vi "Initiate Stream.vi"(0 "niUsrpRio Session":T1={"FPGA Interface"=refnum, "RIO Interface Number"=0, "Data Clock Rate"=0, "FPGA Data Clock Rate"=0, "Global Settings Register Bus"=refnum, "Radio 0 Settings Register Bus"=refnum, "Radio 1 Settings Register Bus"=refnum, "Radio Settings Bus Semaphore"=refnum, "DB Queues"=[], "Characterization Data Valid?"=FALSE, "EEPROM Header"={"Checksum"=0, "Product Code"=0, "Hardware Current Version"=0, "Hardware Oldest Compatible Version"=0, "EEPROM Map Current Version"=0, "EEPROM Map Oldest Compatible Version"=0, "User Password"="", "Pointer to Factory Header"=0, "Pointer to User Header"=0, "Recommended Interval"=0, "Number of Reserved Bytes"=9, "Number of Daughterboards"=0, "Daughterboard IDs"=[], "Daughterboard Serial Numbers"=[]}, "Device Data Header"={"Checksum"=0, "Number of Channels"=0, "Number of Gain Settings"=[], "Pointer to Characterization Data"=[], "Number of Reserved Bytes"=27, "Number of Frequencies"=[]}, "EEPROM Characterization Header"={"Checksum"=0, "Date"=timestamp(0 s since 1904-01-01), "Temperature"=0.0, "Misc. Info"="", "Pointer to Device Data Header"=0, "Number of Reserved Bytes"=28}, "Characterization Data"=[], "FPGA Current Version"=0, "FPGA Oldest Compatible Version"=0, "Fixed Logic Current Version"=0, "Fixed Logic Oldest Compatible Version"=0, "FPGA Radio Settings Bus Current Version"=0, "FPGA Radio Settings Bus Oldest Compatible Version"=0, "FPGA Board Config Current Version"=0, "FPGA Board Config Oldest Compatible Version"=0, "Daughterboard Clock Rate"=0, "daughterboard configuration session handles"=[]} {"Daughterboard Clock Rate" format="%#.3pHz"; "FPGA Data Clock Rate" format="%#.3pHz"; "Data Clock Rate" format="%#.3pHz"; "Characterization Data"."Frequencies [Hz]" format="%#_6p"; "EEPROM Characterization Header"."Pointer to Device Data Header" format="%x"; "EEPROM Characterization Header"."Checksum" format="%x"; "Device Data Header"."Pointer to Characterization Data" format="%x"; "Device Data Header"."Checksum" format="%x"; "EEPROM Header"."Pointer to User Header" format="%x"; "EEPROM Header"."Pointer to Factory Header" format="%x"; "EEPROM Header"."Product Code" format="%x"; "EEPROM Header"."Checksum" format="%x"}, 1 "scope":string(combo)="rx", 11 "error in":errorcluster) -> (4 "niUsrpRio Session (out)":T1={"FPGA Interface"=refnum, "RIO Interface Number"=0, "Data Clock Rate"=0, "FPGA Data Clock Rate"=0, "Global Settings Register Bus"=refnum, "Radio 0 Settings Register Bus"=refnum, "Radio 1 Settings Register Bus"=refnum, "Radio Settings Bus Semaphore"=refnum, "DB Queues"=[], "Characterization Data Valid?"=FALSE, "EEPROM Header"={"Checksum"=0, "Product Code"=0, "Hardware Current Version"=0, "Hardware Oldest Compatible Version"=0, "EEPROM Map Current Version"=0, "EEPROM Map Oldest Compatible Version"=0, "User Password"="", "Pointer to Factory Header"=0, "Pointer to User Header"=0, "Recommended Interval"=0, "Number of Reserved Bytes"=9, "Number of Daughterboards"=0, "Daughterboard IDs"=[], "Daughterboard Serial Numbers"=[]}, "Device Data Header"={"Checksum"=0, "Number of Channels"=0, "Number of Gain Settings"=[], "Pointer to Characterization Data"=[], "Number of Reserved Bytes"=27, "Number of Frequencies"=[]}, "EEPROM Characterization Header"={"Checksum"=0, "Date"=timestamp(0 s since 1904-01-01), "Temperature"=0.0, "Misc. Info"="", "Pointer to Device Data Header"=0, "Number of Reserved Bytes"=28}, "Characterization Data"=[], "FPGA Current Version"=0, "FPGA Oldest Compatible Version"=0, "Fixed Logic Current Version"=0, "Fixed Logic Oldest Compatible Version"=0, "FPGA Radio Settings Bus Current Version"=0, "FPGA Radio Settings Bus Oldest Compatible Version"=0, "FPGA Board Config Current Version"=0, "FPGA Board Config Oldest Compatible Version"=0, "Daughterboard Clock Rate"=0, "daughterboard configuration session handles"=[]} {"Daughterboard Clock Rate" format="%#.3pHz"; "FPGA Data Clock Rate" format="%#.3pHz"; "Data Clock Rate" format="%#.3pHz"; "Characterization Data"."Frequencies [Hz]" format="%#_6p"; "EEPROM Characterization Header"."Pointer to Device Data Header" format="%x"; "EEPROM Characterization Header"."Checksum" format="%x"; "Device Data Header"."Pointer to Characterization Data" format="%x"; "Device Data Header"."Checksum" format="%x"; "EEPROM Header"."Pointer to User Header" format="%x"; "EEPROM Header"."Pointer to Factory Header" format="%x"; "EEPROM Header"."Product Code" format="%x"; "EEPROM Header"."Checksum" format="%x"}, 15 "error out":errorcluster)   [LabVIEW 2020]
doc: "Initiates the stream. This is required before you acquire/generate data with the Fetch Rx Data or Write Tx Data VIs. Initiation includes resetting the Rx/Tx streams and the DSP.\n\n<b>Multi-device usage:</b>\nInitiate the master device last, after initiating all the slave devices.\n\n<B>Input Parameters</B>\n\n<B>niUsrpRio Session</B> is the object created by the Open VI and used as the session handle for the USRP RIO design library.\n\n<B>scope</B> is the channel on which stream is to be initiated. The options are \"rx/RF 0\", \"rx/RF 1\", \"tx/RF 0\", and \"tx/RF 1\".\n\n<B>error in</B> describes error conditions that occur before this node runs. This input provides standard 'error in' functionality.\n\n<B>Output Parameters</B>\n\n<B>niUsrpRio Session (out)</B> is the niUsrpRio session used in all subsequent USRP RIO design library host VIs.\n\n<B>error out</B> contains error information. This output provides standard 'error out' functionality."
uses:
  <instrlib>/niUsrpRio/Config/v1/Host/Public/niUsrpRio Session.ctl
  <instrlib>/_niInstr/Register Bus/v0/Host/Public/Register Bus Session.ctl
  <instrlib>/_niInstr/Register Bus/v0/Host/Private/Session Data.ctl
  <instrlib>/niUsrpRio/Config/v1/Host/Private/DB Queue Reference.ctl
  <instrlib>/niUsrpRio/Config/v1/Host/Private/Daughterboard Data.ctl
  <instrlib>/niUsrpRio/Config/v1/Host/Private/ATR state data.ctl
  <instrlib>/niUsrpRio/Config/v1/Host/Private/Antenna Configuration.ctl
  <instrlib>/niUsrpRio/Config/v1/Host/Private/CPLD Power Mode.ctl
  <instrlib>/niUsrpRio/Config/v1/Host/Public/EEPROM Header.ctl
  <instrlib>/niUsrpRio/Config/v1/Host/Public/EEPROM Device Data Header.ctl
  <instrlib>/niUsrpRio/Config/v1/Host/Public/EEPROM Characterization Header.ctl
  <instrlib>/niUsrpRio/Config/v1/Host/Public/Characterization Data.ctl
  <instrlib>/niUsrpRio/Config/v1/Host/Public/IQ Imbalance.ctl
  Streaming Xvcr FPGA Ref.ctl
  <vilib>/Utility/error.llb/Error Cluster From Error Code.vi
  <vilib>/rvi/errors/niLvFpgaAdjustHostInterfaceError.vi
  <vilib>/ErrorRing/Error Ring.xnode
  <vilib>/rvi/interface/nirviReadWriteControl/nirviReadWriteControl.xnode
  <vilib>/rvi/interface/Simulation/niFpgaSimulationCallBeginRW.vi
  NiFpgaLv.dll
  <instrlib>/niUsrpRio/Config/v1/Host/niUsrpRio Config v1 Host.lvlib
  <instrlib>/_niInstr/Register Bus/v0/Host/niInstr Register Bus v0 Host.lvlib
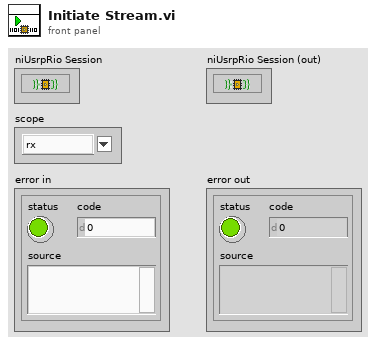
[diagram p1: front panel]
types:
  T1 = typedef "niUsrpRio Config v1 Host.lvlib/niUsrpRio Session.ctl" = cluster{"FPGA Interface":refnum<k20>, "RIO Interface Number":u32, "Data Clock Rate":u32, "FPGA Data Clock Rate":u32, "Global Settings Register Bus":T2, "Radio 0 Settings Register Bus":T2, "Radio 1 Settings Register Bus":T2, "Radio Settings Bus Semaphore":T3, "DB Queues":T4[], "Characterization Data Valid?":bool, "EEPROM Header":T5, "Device Data Header":T6, "EEPROM Characterization Header":T7, "Characterization Data":T8[], "FPGA Current Version":u32, "FPGA Oldest Compatible Version":u32, "Fixed Logic Current Version":u32, "Fixed Logic Oldest Compatible Version":u32, "FPGA Radio Settings Bus Current Version":u32, "FPGA Radio Settings Bus Oldest Compatible Version":u32, "FPGA Board Config Current Version":u32, "FPGA Board Config Oldest Compatible Version":u32, "Daughterboard Clock Rate":u32, "daughterboard configuration session handles":u64[]}
  T2 = typedef "niInstr Register Bus v0 Host.lvlib/Register Bus Session.ctl" = refnum<queue>
  T3 = typedef "Semaphore RefNum" = refnum<k1>
  T4 = typedef "niUsrpRio Config v1 Host.lvlib/DB Queue Reference.ctl" = refnum<queue>
  T5 = typedef "niUsrpRio Config v1 Host.lvlib/EEPROM Header.ctl" = cluster{"Checksum":u32, "Product Code":u16, "Hardware Current Version":u16, "Hardware Oldest Compatible Version":u16, "EEPROM Map Current Version":u16, "EEPROM Map Oldest Compatible Version":u16, "User Password":string, "Pointer to Factory Header":u32, "Pointer to User Header":u32, "Recommended Interval":u16, "Number of Reserved Bytes":i32, "Number of Daughterboards":u8, "Daughterboard IDs":u16[], "Daughterboard Serial Numbers":string[]}
  T6 = typedef "niUsrpRio Config v1 Host.lvlib/EEPROM Device Data Header.ctl" = cluster{"Checksum":u32, "Number of Channels":u8, "Number of Gain Settings":u16[], "Pointer to Characterization Data":u32[], "Number of Reserved Bytes":i32, "Number of Frequencies":u16[]}
  T7 = typedef "niUsrpRio Config v1 Host.lvlib/EEPROM Characterization Header.ctl" = cluster{"Checksum":u32, "Date":timestamp, "Temperature":sgl, "Misc. Info":string, "Pointer to Device Data Header":u32, "Number of Reserved Bytes":i32}
  T8 = typedef "niUsrpRio Config v1 Host.lvlib/Characterization Data.ctl" = cluster{"Gains[dB]":dbl[], "Frequencies [Hz]":dbl[], "IQ Imbalance Table":T9[], "Measured Gains[dB]":dbl[][]}
  T9 = typedef "niUsrpRio Config v1 Host.lvlib/IQ Imbalance.ctl" = cluster{"Gain Imbalance [linear]":dbl, "Phase Imbalance [radians]":dbl, "Offset":cdb}
  T10 = typedef "Streaming Xvcr FPGA Ref.ctl" = refnum<k20>
  T11 = typedef "niUsrpRio Config v1 Host.lvlib/Device Subfunction.ctl" = enum16{"rx", "tx", "all"}
  T12 = typedef "niUsrpRio Config v1 Host.lvlib/RF Channel 2.ctl" = enum16{"0", "1", "2", "3", "All"}
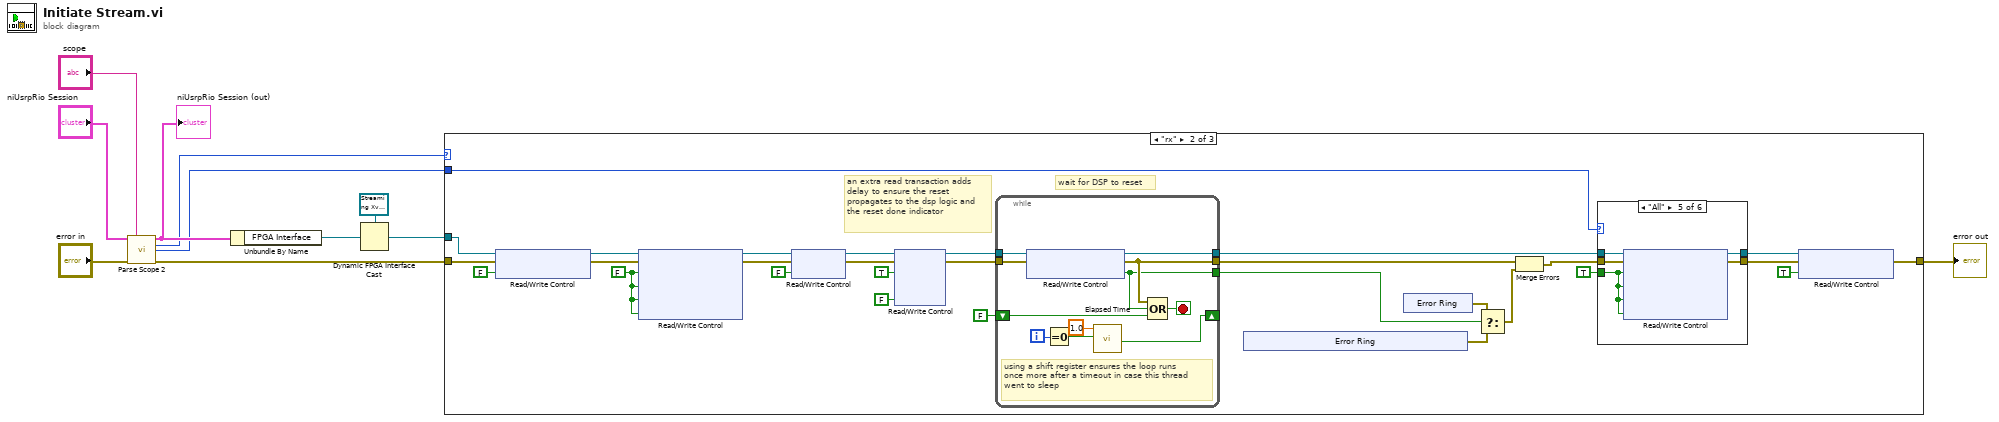
[diagram p0: block diagram]
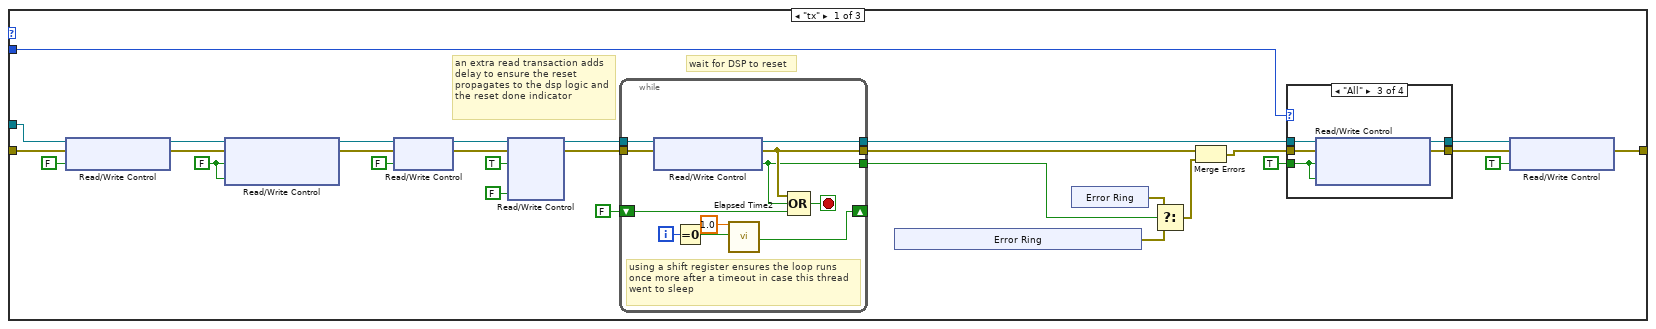
[diagram p2: hidden frame]
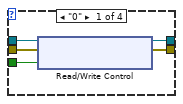
[diagram p3: hidden frame]
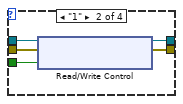
[diagram p4: hidden frame]
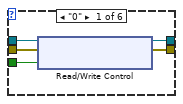
[diagram p6: hidden frame]
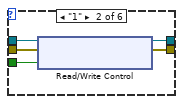
[diagram p7: hidden frame]
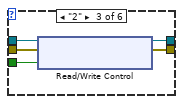
[diagram p8: hidden frame]
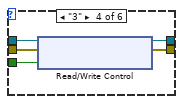
[diagram p9: hidden frame]
diagram:
  n1 = call <instrlib>:"Parse Scope 2.vi"("niUsrpRio Session"="niUsrpRio Session", "scope"="scope", "error in"="error in") -> ("niUsrpRio Session (out)"=w11:T1, "Device Subfunction"=w8:T11, "Device Subfunction Channel"=w7:T12, "error out"=w6:errorcluster)  [unwired: 4 in, 5 out]
  "niUsrpRio Session (out)" <- w11
  n2 = Unbundle By Name(w11) -> ("FPGA Interface"=w4:refnum<k20>)
  n3 = Dynamic FPGA Interface Cast(Session In=T10 refnum ("Type"), Type=w4) -> (Session Out=w3:T10)
  n4 = case shown="\"rx\"" w8 {
    tunnel: w3 -> [w24 w85 _]
    tunnel: [w25 w86 w148] -> w2
    tunnel: w6 -> [w31 w92 w148]
    tunnel: w7 -> [w32 w93 _]
    frame "tx" {
      w12 = FALSE ("tx 0.stream enable")
      # "an extra read transaction adds delay to ensure the reset propagates to the dsp logic and the reset done indicator"
      # "wait for DSP to reset"
      n5 = xnode "Read/Write Control"("FPGA VI Reference In"=w24, "error in"=w31, "tx.trigger enable"=FALSE) -> ("FPGA VI Reference Out"=w29:T10, "error out"=w30:errorcluster)
      n6 = xnode "Read/Write Control"("FPGA VI Reference In"=w29, "error in"=w30, "tx 0.stream enable"=w12, "tx 1.stream enable"=w12) -> ("FPGA VI Reference Out"=w35:T10, "error out"=w36:errorcluster)
      n7 = xnode "Read/Write Control"("FPGA VI Reference In"=w35, "error in"=w36, "tx.abort"=FALSE) -> ("FPGA VI Reference Out"=w18:T10, "error out"=w17:errorcluster)
      n8 = xnode "Read/Write Control"("FPGA VI Reference In"=w18, "error in"=w17, "tx.reset"=TRUE, "tx.reset"=FALSE) -> ("FPGA VI Reference Out"=w14:T10, "error out"=w15:errorcluster)  [unwired: 1 out]
      n9 = while {
        tunnel: [w70] -> w21
        tunnel: [w69] -> w20
        shift-right: [w67] -> _
        shift-left: FALSE ("Time has Elapsed") -> [w68]
        tunnel: [w66] -> w22
        tunnel: w15 -> [w65]
        tunnel: w14 -> [w64]
        i -> [w73]
        stop <- w71 stop-if-true
        # "using a shift register ensures the loop runs once more after a timeout in case this thread went to sleep"
        n10 = xnode "Read/Write Control"("FPGA VI Reference In"=w64, "error in"=w65) -> ("FPGA VI Reference Out"=w69:T10, "error out"=w70:errorcluster, "tx.dsp reset done"=w66:bool)
        n11 = Equal To 0?(x=w73) -> (x = 0?=w74:bool)
        n12 = call "Elapsed Time2"("Time Target (s)"=1.0, "Reset"=w74) -> ("Time has Elapsed"=w67:bool)  [unwired: 10 in, 7 out]
        n13 = Compound Arithmetic op=OR(w70, w66, w68) -> (w71:bool)
      }
      n14 = xnode "Error Ring"() -> ("error out"=w37:errorcluster)
      n15 = xnode "Error Ring"() -> ("error out"=w38:errorcluster)
      n16 = Select(t=w38, s=w22, f=w37) -> (s? t:f=w39:errorcluster)
      n17 = Merge Errors(w21, w39) -> (w33:errorcluster)
      n18 = case shown="\"All\"" w32 {
        tunnel: w33 -> [w45 w50 w55 w57]
        tunnel: w20 -> [w44 w46 w54 w56]
        tunnel: [w43 w48 w53 w57] -> w26
        tunnel: [w42 w49 w52 w56] -> w27
        tunnel: TRUE ("tx.stream enabled") -> [w41 w47 w51 _]
        frame "0" {
          n19 = xnode "Read/Write Control"("FPGA VI Reference In"=w44, "error in"=w45, "tx 0.stream enable"=w41) -> ("FPGA VI Reference Out"=w42:T10, "error out"=w43:errorcluster)
        }
        frame "1" {
          n20 = xnode "Read/Write Control"("FPGA VI Reference In"=w46, "error in"=w50, "tx 1.stream enable"=w47) -> ("FPGA VI Reference Out"=w49:T10, "error out"=w48:errorcluster)
        }
        frame "All" {
          n21 = xnode "Read/Write Control"("FPGA VI Reference In"=w54, "error in"=w55, "tx 0.stream enable"=w51, "tx 1.stream enable"=w51) -> ("FPGA VI Reference Out"=w52:T10, "error out"=w53:errorcluster)
        }
        frame Default {
        }
      }
      n22 = xnode "Read/Write Control"("FPGA VI Reference In"=w27, "error in"=w26, "tx.trigger enable"=TRUE ("tx.enable trigger")) -> ("error out"=w25:errorcluster)  [unwired: 1 out]
    }
    frame "rx" {
      w75 = FALSE ("tx 0.stream enable")
      # "an extra read transaction adds delay to ensure the reset propagates to the dsp logic and the reset done indicator"
      # "wait for DSP to reset"
      n23 = xnode "Read/Write Control"("FPGA VI Reference In"=w85, "error in"=w92, "rx.trigger enable"=FALSE ("tx.trigger enable")) -> ("FPGA VI Reference Out"=w90:T10, "error out"=w91:errorcluster)
      n24 = xnode "Read/Write Control"("FPGA VI Reference In"=w90, "error in"=w91, "rx 0.stream enable"=w75, "rx 1.stream enable"=w75, "rx 2.stream enable"=w75, "rx 3.stream enable"=w75) -> ("FPGA VI Reference Out"=w96:T10, "error out"=w97:errorcluster)
      n25 = xnode "Read/Write Control"("FPGA VI Reference In"=w96, "error in"=w97, "rx.abort"=FALSE ("tx.abort")) -> ("FPGA VI Reference Out"=w101:T10, "error out"=w102:errorcluster)
      n26 = xnode "Read/Write Control"("FPGA VI Reference In"=w101, "error in"=w102, "rx.reset"=TRUE ("tx.reset"), "rx.reset"=FALSE ("tx.reset")) -> ("FPGA VI Reference Out"=w76:T10, "error out"=w77:errorcluster)  [unwired: 1 out]
      n27 = while {
        tunnel: w76 -> [w147]
        tunnel: w77 -> [w146]
        tunnel: [w141] -> w82
        tunnel: [w140] -> w81
        shift-right: [w138] -> _
        shift-left: FALSE ("Time has Elapsed") -> [w139]
        tunnel: [w137] -> w83
        i -> [w144]
        stop <- w142 stop-if-true
        # "using a shift register ensures the loop runs once more after a timeout in case this thread went to sleep"
        n28 = xnode "Read/Write Control"("FPGA VI Reference In"=w147, "error in"=w146) -> ("FPGA VI Reference Out"=w140:T10, "error out"=w141:errorcluster, "rx.dsp reset done"=w137:bool)
        n29 = Equal To 0?(x=w144) -> (x = 0?=w145:bool)
        n30 = call "Elapsed Time"("Time Target (s)"=1.0, "Reset"=w145) -> ("Time has Elapsed"=w138:bool)  [unwired: 10 in, 7 out]
        n31 = Compound Arithmetic op=OR(w141, w137, w139) -> (w142:bool)
      }
      n32 = xnode "Error Ring"() -> ("error out"=w98:errorcluster)
      n33 = xnode "Error Ring"() -> ("error out"=w99:errorcluster)
      n34 = Select(t=w99, s=w83, f=w98) -> (s? t:f=w100:errorcluster)
      n35 = Merge Errors(w82, w100) -> (w94:errorcluster)
      n36 = case shown="\"All\"" w93 {
        tunnel: w94 -> [w108 w113 w118 w123 w128 w130]
        tunnel: w81 -> [w107 w109 w114 w122 w127 w129]
        tunnel: [w106 w111 w116 w121 w126 w130] -> w87
        tunnel: [w105 w112 w117 w120 w125 w129] -> w88
        tunnel: TRUE ("tx.stream enabled") -> [w104 w110 w115 w119 w124 _]
        frame "0" {
          n37 = xnode "Read/Write Control"("FPGA VI Reference In"=w107, "error in"=w108, "rx 0.stream enable"=w104) -> ("FPGA VI Reference Out"=w105:T10, "error out"=w106:errorcluster)
        }
        frame "1" {
          n38 = xnode "Read/Write Control"("FPGA VI Reference In"=w109, "error in"=w113, "rx 1.stream enable"=w110) -> ("FPGA VI Reference Out"=w112:T10, "error out"=w111:errorcluster)
        }
        frame "2" {
          n39 = xnode "Read/Write Control"("FPGA VI Reference In"=w114, "error in"=w118, "rx 2.stream enable"=w115) -> ("FPGA VI Reference Out"=w117:T10, "error out"=w116:errorcluster)
        }
        frame "3" {
          n40 = xnode "Read/Write Control"("FPGA VI Reference In"=w122, "error in"=w123, "rx 3.stream enable"=w119) -> ("FPGA VI Reference Out"=w120:T10, "error out"=w121:errorcluster)
        }
        frame "All" {
          n41 = xnode "Read/Write Control"("FPGA VI Reference In"=w127, "error in"=w128, "rx 0.stream enable"=w124, "rx 1.stream enable"=w124, "rx 2.stream enable"=w124, "rx 3.stream enable"=w124) -> ("FPGA VI Reference Out"=w125:T10, "error out"=w126:errorcluster)
        }
        frame Default {
        }
      }
      n42 = xnode "Read/Write Control"("FPGA VI Reference In"=w88, "error in"=w87, "rx.trigger enable"=TRUE ("tx.enable trigger")) -> ("error out"=w86:errorcluster)  [unwired: 1 out]
    }
    frame Default {
    }
  }
  "error out" <- w2
